vi "6.6.vi"() -> ()   [LabVIEW 2017]
panel:
  out "字符串":string
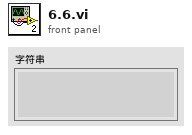
[diagram p1: front panel]
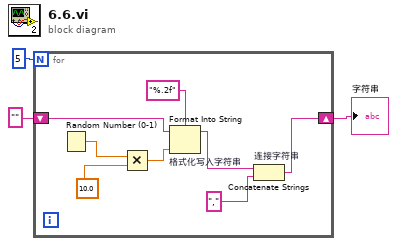
[diagram p0: block diagram]
diagram:
  n1 = for {
    N: 5 -> [_]
    shift-right: [w5] -> w1
    shift-left: "" -> [w4]
    n2 = Random Number (0-1)() -> (number: 0 to 1=w11:dbl)
    n3 = Multiply(x=w11, y=10.0) -> (x*y=w8:dbl)
    n4 = Format Into String "格式化写入字符串"(format string="%.2f", initial string=w4, w8) -> (resulting string=w10:string)  [unwired: 1 in, 1 out]
    n5 = Concatenate Strings "连接字符串"(w10, ",") -> (w5:string)
  }
  "字符串" <- w1
